vi "GEOM_FPAamplifiersList.vi"(8 "error in (no error)":errorcluster, 9 "FPAReadMode":T7={"name"="", "Read Type"="interleaved", "ReadModes"=[]}, 10 "Detectors":T8 {"ReadModes"."amplifiers"."fliped" items=["none", "horizontal", "vertical"]; "ReadModes"."amplifiers"."type" items=["LL", "LR", "UL", "UR"]}) -> (0 "error out":errorcluster, 1 "detreadmode":cluster{"name":string, "detectors":T1[]}, 2 "FPAReadMode 2":T2 {"Amplifiers"."fliped" items=["none", "horizontal", "vertical"]; "Amplifiers"."type" items=["LL", "LR", "UL", "UR"]})   [LabVIEW 2016]
uses:
  GEOM_FPADetectors.ctl
  GEOM_DetStruct.ctl
  GEOM_ReadMode.ctl
  GEOM_Amplifier.ctl
  GEOM_AmpType.ctl
  GEOM_ROI.ctl
  GEOM_Coords.ctl
  GEOM_FPAReadMode.ctl
  GEOM_DetSummaryStruct.ctl
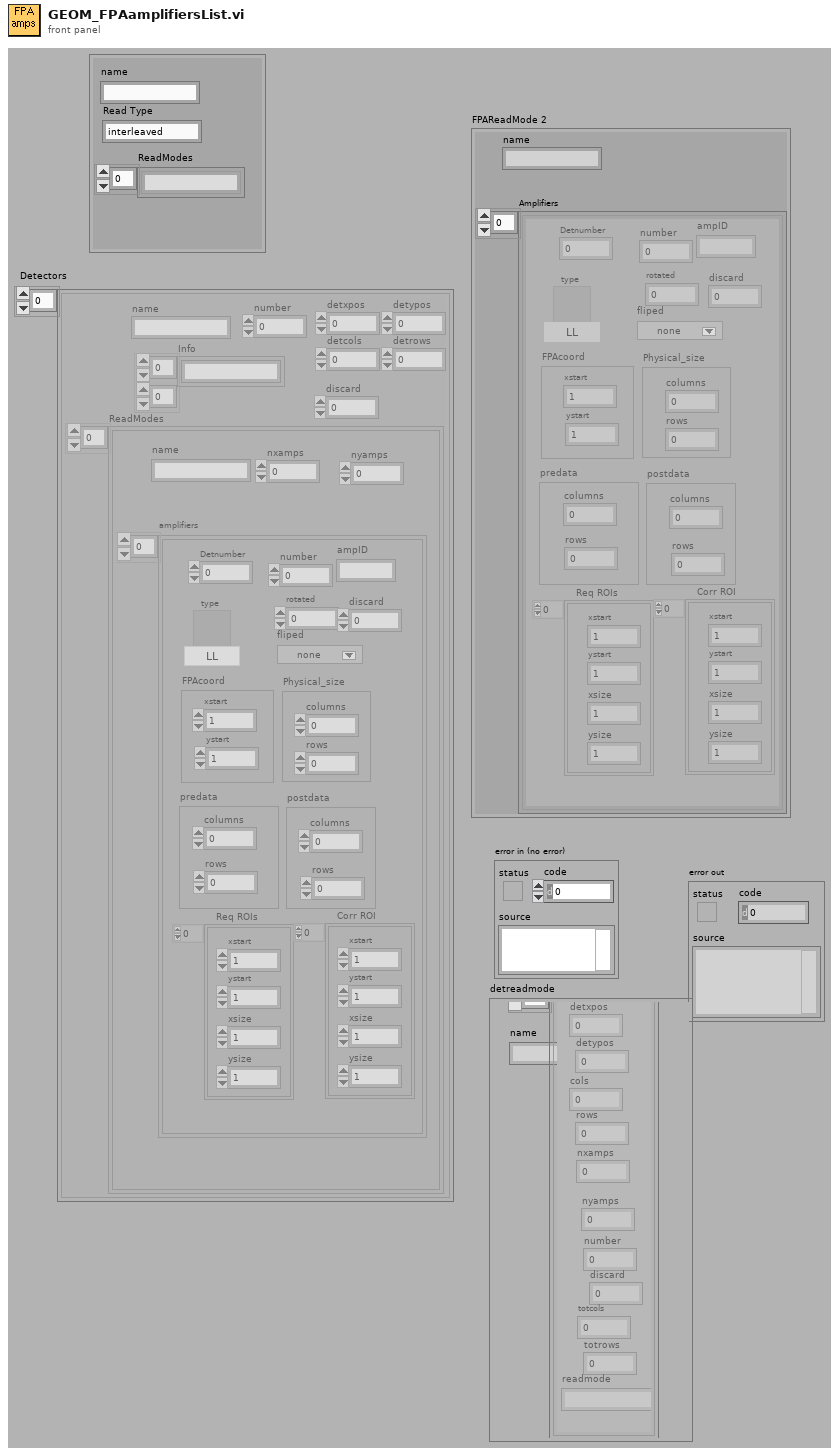
[diagram p1: front panel]
types:
  T1 = typedef "GEOM_DetSummaryStruct.ctl" = cluster{"detxpos":i32, "detypos":i32, "cols":i32, "rows":i32, "nxamps":i32, "nyamps":i32, "number":i32, "discard":i32, "totcols":i32, "totrows":i32, "readmode":string}
  T2 = typedef "GEOM_FPAReadMode.ctl" = cluster{"name":string, "Amplifiers":T3[]}
  T3 = typedef "GEOM_Amplifier.ctl" = cluster{"number":i32, "type":T4, "rotated":i16, "fliped":u16, "FPAcoord":cluster{"xstart":i32, "ystart":i32}, "Physical_size":cluster{"columns":i32, "rows":i32}, "predata":cluster{"columns":i32, "rows":i32}, "postdata":cluster{"columns":i32, "rows":i32}, "Req ROIs":T5, "Corr ROI":T5, "Detnumber":i32, "ampID":string, "discard":i32}
  T4 = typedef "GEOM_AmpType.ctl" = u16
  T5 = typedef "GEOM_ROI.ctl" = T6[]
  T6 = typedef "GEOM_Coords.ctl" = cluster{"xstart":u32, "ystart":u32, "xsize":u32, "ysize":u32}
  T7 = cluster{"name":string, "Read Type":string, "ReadModes":string[]}
  T8 = typedef "GEOM_FPADetectors.ctl" = T9[]
  T9 = typedef "GEOM_DetStruct.ctl" = cluster{"name":string, "number":i32, "Info":string[][], "ReadModes":T10[], "detxpos":i32, "detypos":i32, "detcols":i32, "detrows":i32, "discard":i32}
  T10 = typedef "GEOM_ReadMode.ctl" = cluster{"name":string, "amplifiers":T3[], "nxamps":i32, "nyamps":i32}
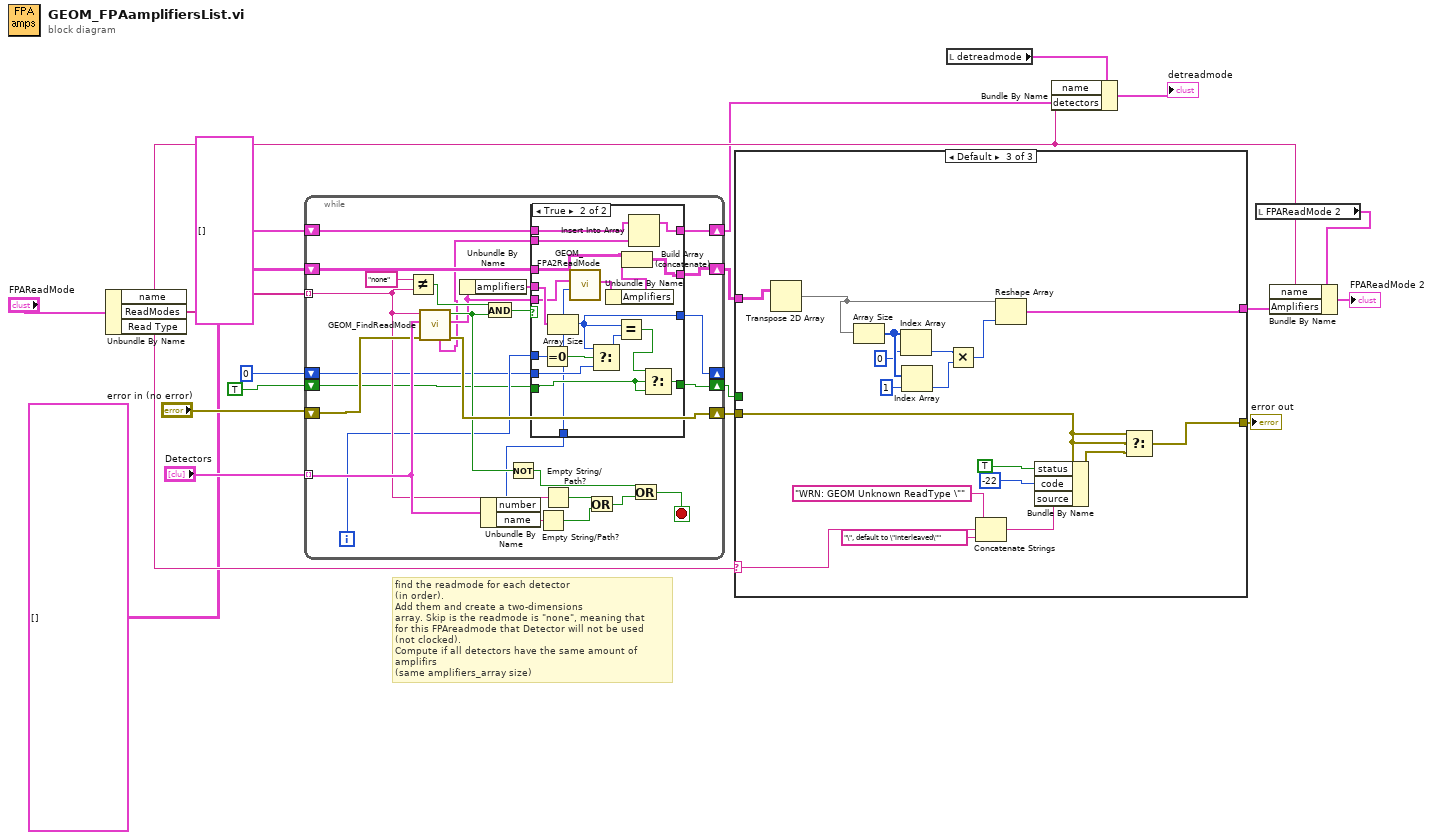
[diagram p0: block diagram]
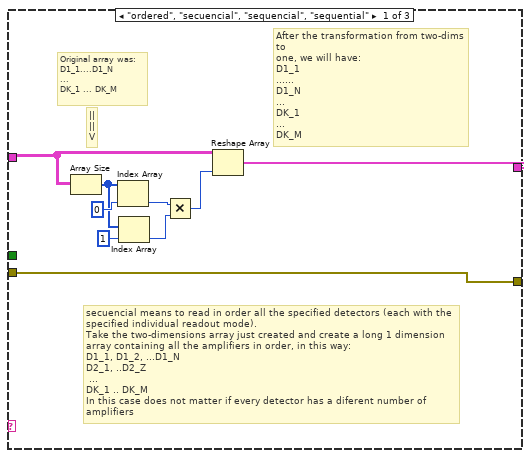
[diagram p3: hidden frame]
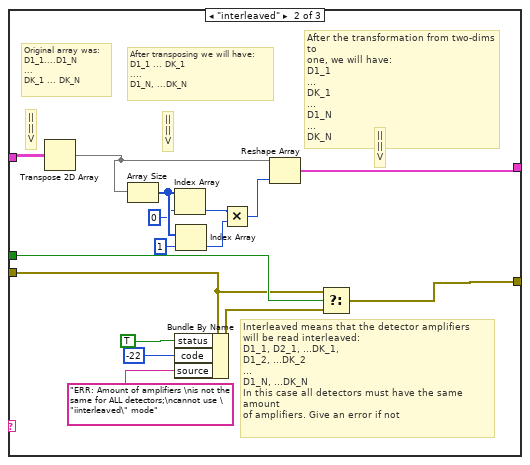
[diagram p4: hidden frame]
diagram:
  # "find the readmode for each detector\n(in order). \nAdd them and create a two-dimensions\narray. Skip is the readmode is \"none\", meaning that\nfor this FPAreadmode that Detector will not be used\n(not clocked).\nCompute if all detectors have the same amount of amplifirs\n(same amplifiers_array size)"
  n1 = Unbundle By Name("FPAReadMode") -> ("name"=w3:string, "ReadModes"=w1:string[], "Read Type"=w19:string)
  n2 = while {
    tunnel: "Detectors" -> [w46] mode=indexing
    tunnel: w1 -> [w37] mode=indexing
    shift-right: [w26] -> w10
    shift-left: T3[][] [] -> [w25]
    shift-right: [w39] -> w15
    shift-left: "error in (no error)" -> [w40]
    shift-right: [w30] -> _
    shift-left: 0 -> [w31]
    shift-right: [w29] -> w11
    shift-left: TRUE -> [w28]
    shift-right: [w23] -> w2
    shift-left: T1[] [] -> [w22]
    i -> [w32]
    stop <- w47 stop-if-true
    n3 = Not Equal?(x="none", y=w37) -> (x != y?=w35:bool)
    n4 = call "GEOM_FindReadMode.vi"("error in (no error)"=w40, "Detector"=w46, "ReadMode name"=w37) -> ("error out"=w39:errorcluster, "ReadMode"=w27:T10, "found?"=w38:bool, "detector"=w21:T1)  [unwired: 5 out]
    n5 = Unbundle By Name(w27) -> ("amplifiers"=w33:T3[])
    n6 = Unbundle By Name(w46) -> ("number"=w24:i32, "name"=w45:string)
    n7 = And(x=w35, y=w38) -> (x .and. y?=w34:bool)
    n8 = Not(x=w38) -> (.not. x?=w41:bool)
    n9 = case shown="True" w34 {
      tunnel: w33 -> [_ w61]
      tunnel: [w49 w60] -> w26
      tunnel: w32 -> [_ w69]
      tunnel: w31 -> [w51 w66]
      tunnel: [w50 w62] -> w29
      tunnel: [w51 w65] -> w30
      tunnel: w28 -> [w50 w63]
      tunnel: w27 -> [_ w55]
      tunnel: w25 -> [w49 w59]
      tunnel: w24 -> [_ w56]
      tunnel: [w48 w54] -> w23
      tunnel: w22 -> [w48 w53]
      tunnel: w21 -> [_ w52]
      frame False {
      }
      frame True {
        n10 = Equal To 0?(x=w69) -> (x = 0?=w68:bool)
        n11 = Array Size(array=w61) -> (size(s)=w65:i32)
        n12 = call "GEOM_FPA2ReadMode.vi"("Detnumber"=w56, "ReadMode"=w55) -> ("output ReadMode"=w58:T2)  [unwired: 9 out]
        n13 = Select(t=w65, s=w68, f=w66) -> (s? t:f=w67:i32)
        n14 = Unbundle By Name(w58) -> ("Amplifiers"=w57:T3[])
        n15 = Equal?(x=w65, y=w67) -> (x = y?=w64:bool)
        n16 = Build Array (concatenate)(w59, w57) -> (w60:T3[][])
        n17 = Insert Into Array(array=w53, new element=w52) -> (w54:T1[])  [unwired: 1 in]
        n18 = Select(t=w64, s=w63, f=w63) -> (s? t:f=w62:bool)
      }
    }
    n19 = Empty String/Path?(string/path=w45) -> (empty?=w44:bool)
    n20 = Empty String/Path?(string/path=w37) -> (empty?=w43:bool)
    n21 = Or(x=w43, y=w44) -> (x .or. y?=w42:bool)
    n22 = Or(x=w41, y=w42) -> (x .or. y?=w47:bool)
  }
  n23 = case shown="Default" w19 {
    selector: w19 -> [_ _ w99]
    tunnel: [w75 w79 w95] -> w17
    tunnel: w15 -> [w74 w85 w104]
    tunnel: [w74 w86 w105] -> w14
    tunnel: w11 -> [_ w87 _]
    tunnel: w10 -> [w73 w80 w96]
    frame "ordered", "secuencial", "sequencial", "sequential" {
      # "After the transformation from two-dims to\none, we will have:\nD1_1\n......\nD1_N\n...\nDK_1\n...\nDK_M"
      # "||\n||\nV"
      # "Original array was:\nD1_1....D1_N\n...\nDK_1 ... DK_M"
      # "secuencial means to read in order all the specified detectors (each with the\nspecified individual readout mode).\nTake the two-dimensions array just created and create a long 1 dimension\narray containing all the amplifiers in order, in this way:\nD1_1, D1_2, ...D1_N\nD2_1, ..D2_Z\n ...\nDK_1 .. DK_M\nIn this case does not matter if every detector has a diferent number of amplifiers"
      n24 = Array Size(array=w73) -> (size(s)=w72:i32[])
      n25 = Index Array(array=w72, index=0) -> (element=w71:i32)
      n26 = Index Array(array=w72, index=1) -> (element=w70:i32)
      n27 = Multiply(x=w71, y=w70) -> (x*y=w76:i32)
      n28 = Reshape Array(w73, w76) -> (w75:T3[])
    }
    frame "interleaved" {
      # "||\n||\nV"
      # "||\n||\nV"
      # "||\n||\nV"
      # "After the transformation from two-dims to\none, we will have:\nD1_1\n...\nDK_1\n...\nD1_N\n...\nDK_N"
      # "After transposing we will have:\nD1_1 ... DK_1\n....\nD1_N, ...DK_N"
      # "Original array was:\nD1_1....D1_N\n...\nDK_1 ... DK_N"
      # "Interleaved means that the detector amplifiers\nwill be read interleaved:\nD1_1, D2_1, ...DK_1, \nD1_2, ...DK_2 \n...\nD1_N, ...DK_N\nIn this case all detectors must have the same amount\nof amplifiers. Give an error if not"
      n29 = Transpose 2D Array(2D array=w80) -> (transposed array=w88:T3[][])
      n30 = Array Size(array=w88) -> (size(s)=w94:i32[])
      n31 = Index Array(array=w94, index=0) -> (element=w91:i32)
      n32 = Bundle By Name(cluster=w85, "status"=TRUE, "code"=-22, "source"="ERR: Amount of amplifiers \nis not the same for ALL detectors;\ncannot use \"iinterleaved\" mode") -> (w84:errorcluster)
      n33 = Index Array(array=w94, index=1) -> (element=w90:i32)
      n34 = Multiply(x=w91, y=w90) -> (x*y=w89:i32)
      n35 = Reshape Array(w88, w89) -> (w79:T3[])
      n36 = Select(t=w85, s=w87, f=w84) -> (s? t:f=w86:errorcluster)
    }
    frame Default {
      n37 = Transpose 2D Array(2D array=w96) -> (transposed array=w106:T3[][])
      n38 = Array Size(array=w106) -> (size(s)=w112:i32[])
      n39 = Index Array(array=w112, index=0) -> (element=w109:i32)
      n40 = Index Array(array=w112, index=1) -> (element=w108:i32)
      n41 = Multiply(x=w109, y=w108) -> (x*y=w107:i32)
      n42 = Concatenate Strings("WRN: GEOM Unknown ReadType \"" ("source"), w99, "\", default to \"interleaved\"" ("string")) -> (w97:string)
      n43 = Reshape Array(w106, w107) -> (w95:T3[])
      n44 = Bundle By Name(cluster=w104, "status"=TRUE, "code"=-22, "source"=w97) -> (w103:errorcluster)
      n45 = Select(t=w104, s=w104, f=w103) -> (s? t:f=w105:errorcluster)
    }
  }
  "error out" <- w14
  n46 = local read "detreadmode"() -> (w5:cluster{"name":string, "detectors":T1[]})
  n47 = Bundle By Name(cluster=w5, "name"=w3, "detectors"=w2) -> (→"detreadmode":cluster{"name":string, "detectors":T1[]})
  n48 = local read "FPAReadMode 2"() -> (w8:T2)
  n49 = Bundle By Name(cluster=w8, "name"=w3, "Amplifiers"=w17) -> (→"FPAReadMode 2":T2)
